vi "Run Service.vi"   [LabVIEW 2020, in "MeasurementLink Measurement Template.lvlib"]
uses:
  MeasurementLink Measurement Template.lvlib
  MeasurementLink Measurement Server/MeasurementLink Measurement Server.lvlib
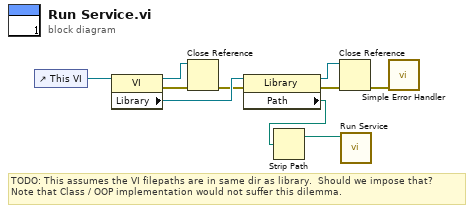
[diagram p0: block diagram]
diagram:
  # "TODO: This assumes the VI filepaths are in same dir as library.  Should we impose that?\nNote that Class / OOP implementation would not suffer this dilemma."
  n1 = control-ref of="This VI"() -> (w10:refnum<vi>)
  n2 = property class="VI"(reference=w10) -> (reference out=w8:refnum<vi>, error out=w9:errorcluster, "Library"=w7:refnum<vi>)  [unwired: 1 in]
  n3 = Close Reference(reference=w8, error in (no error)=w9) -> (error out=w6:errorcluster)
  n4 = property class="Library"(reference=w7, error in=w6) -> (reference out=w4:refnum<vi>, error out=w5:errorcluster, "Path"=w2:path)
  n5 = Strip Path(path=w2) -> (stripped path=w1:path)  [unwired: 1 out]
  n6 = Close Reference(reference=w4, error in (no error)=w5) -> (error out=w3:errorcluster)
  n7 = call "Run Service.vi"("Library Root"=w1) -> ()  [unwired: 11 in]
  n8 = call <vilib>:"Simple Error Handler.vi"("error in (no error)"=w3) -> ()  [unwired: 4 in, 5 out]
